vi "Test Read Axes.vi"() -> ()   [LabVIEW 2013]
doc: "This VI tests reading the axis encoders for the translation table."
uses:
  Controls/table_axis_enum.ctl
panel:
  out "Spike Filtered":bool[](array[boolean])
  out "Position Chart":T1(graph)
  out "Positions Array":dbl[](array[numeric])
  in  "Stop Button":bool
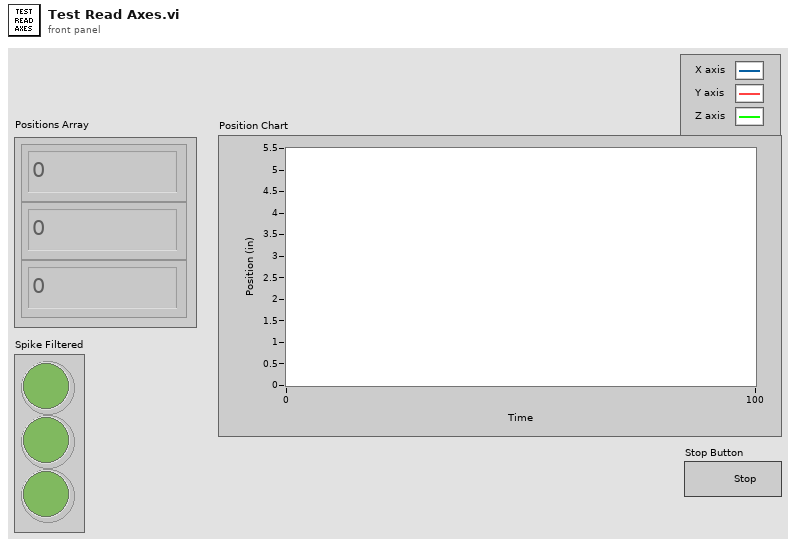
[diagram p1: front panel]
types:
  T1 = cluster{"[0]":dbl, "[1]":dbl, "[2]":dbl, "[3]":dbl, "[4]":dbl, "[5]":dbl, "[6]":dbl, "[7]":dbl, "[8]":dbl}
  T2 = typedef "table_axis_enum.ctl" = enum16{"X-axis", "Y-axis", "Z-axis", "W-axis"}
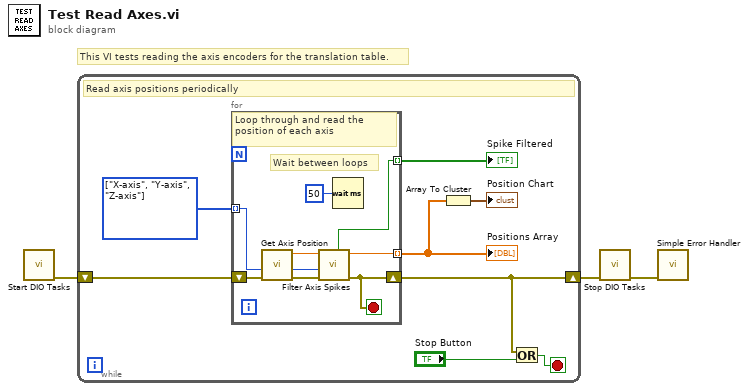
[diagram p0: block diagram]
diagram:
  # "This VI tests reading the axis encoders for the translation table."
  n1 = call "Start DIO Tasks.vi"() -> ("error out"=w3:errorcluster)  [unwired: 11 in]
  n2 = while {
    shift-right: [w10] -> w2
    shift-left: w3 -> [w7]
    stop <- w8 stop-if-true
    w11 = T2[] [enum."X-axis", enum."Y-axis", enum."Z-axis"] items=["X-axis", "Y-axis", "Z-axis", "W-axis"]
    # "Read axis positions periodically"
    n3 = for {
      tunnel: w11 -> [w20] mode=indexing
      shift-right: [w16] -> w10
      shift-left: w7 -> [w19]
      tunnel: [w13] -> w6 mode=indexing
      tunnel: [w12] -> w4 mode=indexing
      stop <- w16 stop-if-true
      # "Wait between loops"
      # "Loop through and read the position of each axis"
      n4 = call "Get Axis Position.vi"("Error In"=w19, "Axis Enum"=w20) -> ("Error Out"=w17:errorcluster, "Axis Enum Out"=w15:T2, "Axis Inches"=w14:dbl)  [unwired: 6 in, 1 out]
      n5 = call "Filter Axis Spikes.vi"("Error In"=w17, "Axis Enum"=w15, "Current Reading"=w14) -> ("Error Out"=w16:errorcluster, "Filtered Reading"=w13:dbl, "Peak Detected?"=w12:bool)  [unwired: 5 in, 1 out]
      n6 = Wait (ms)(milliseconds to wait=u32 50) -> ()  [unwired: 1 out]
    }
    "Positions Array" <- w6
    "Spike Filtered" <- w4
    n7 = Array To Cluster(array=w6) -> (cluster=→"Position Chart":T1)
    n8 = Or(x=w10, y="Stop Button") -> (x .or. y?=w8:bool)
  }
  n9 = call "Stop DIO Tasks.vi"("Error In"=w2) -> ("error out"=w1:errorcluster)  [unwired: 10 in]
  n10 = call <vilib>:"Simple Error Handler.vi"("error in (no error)"=w1) -> ()  [unwired: 4 in, 5 out]
